vi "GraphWindowGen.vi"() -> (11 "XY Graph":cluster{dbl, dbl}[](graph))   [LabVIEW 2010]
panel:
  out "error out":errorcluster caption="sortie d'erreur"
  in  "error in (no error)":errorcluster
  in  "stop":bool
  in  "ToolsVis":bool=TRUE
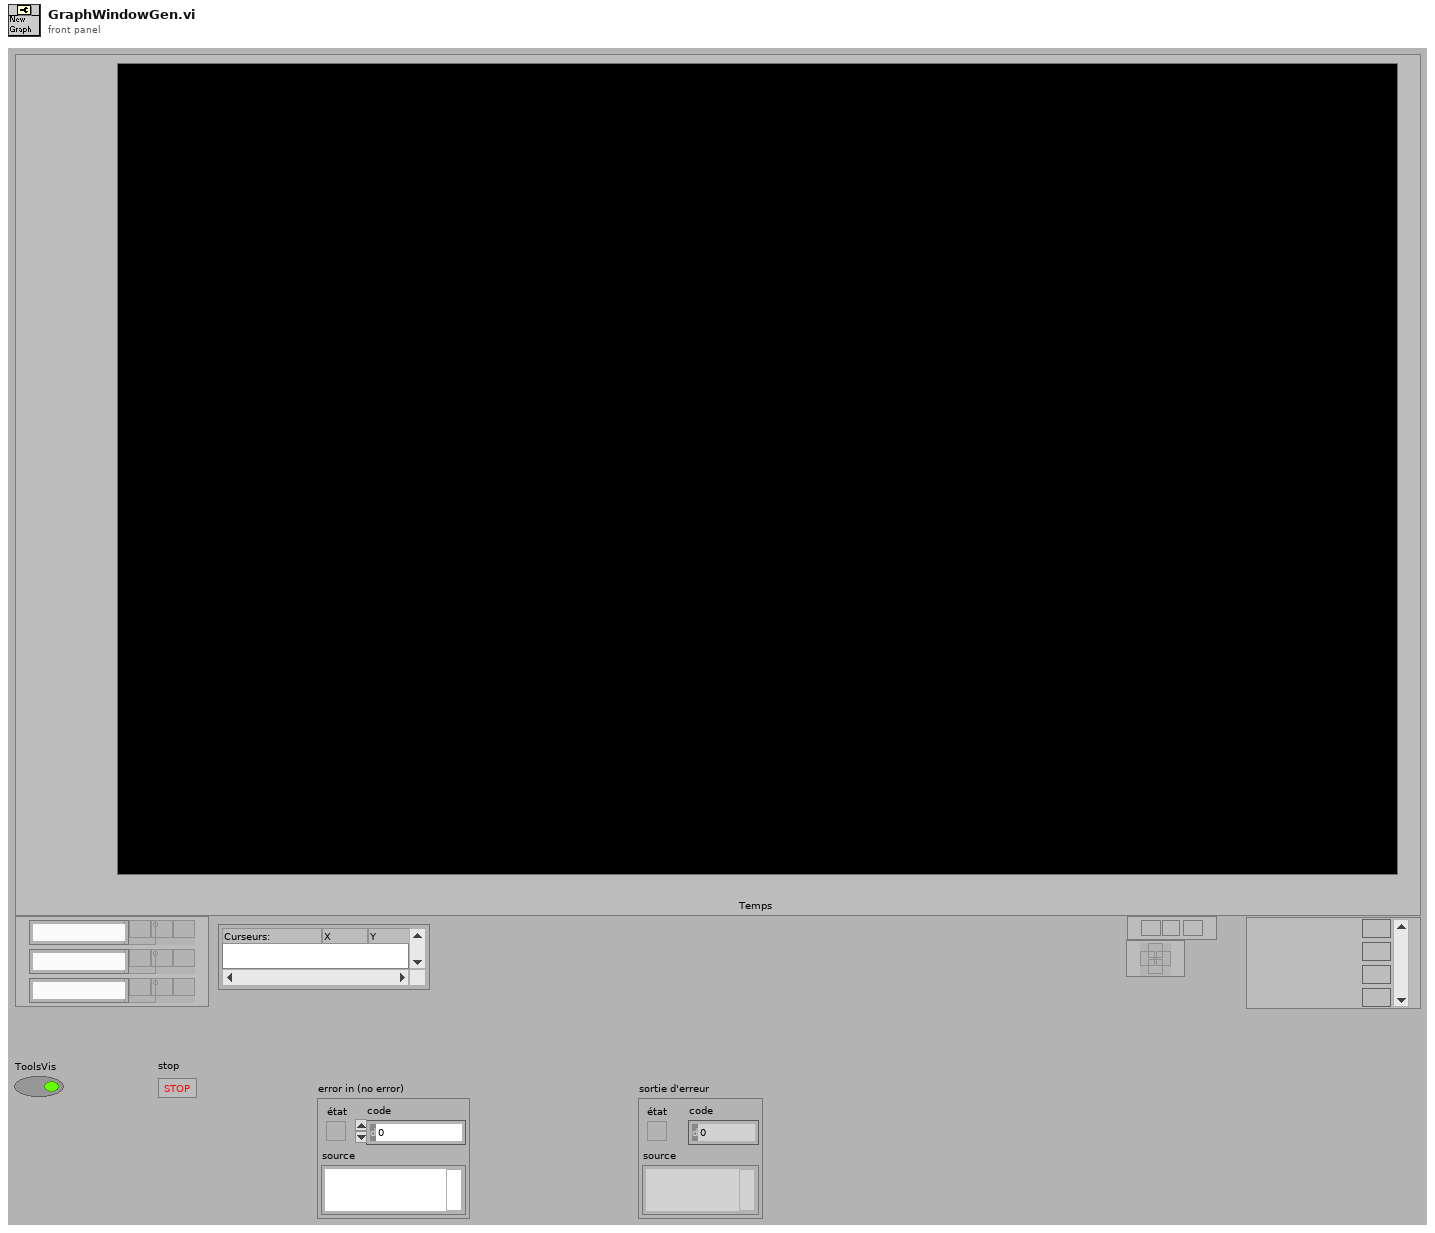
[diagram p1: front panel]
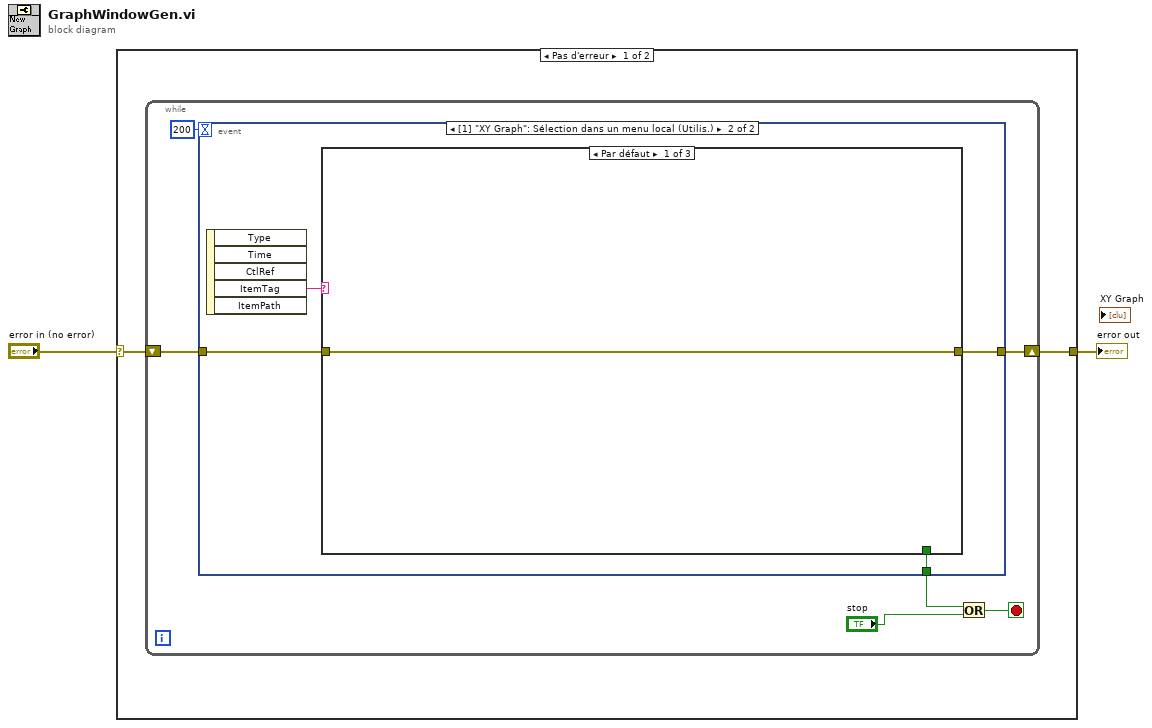
[diagram p0: block diagram]
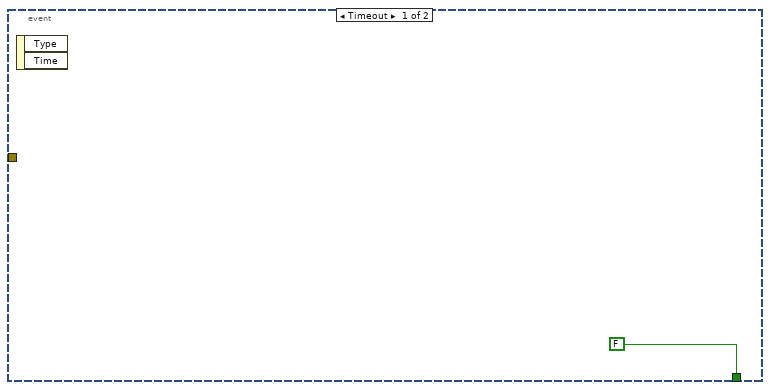
[diagram p2: hidden frame]
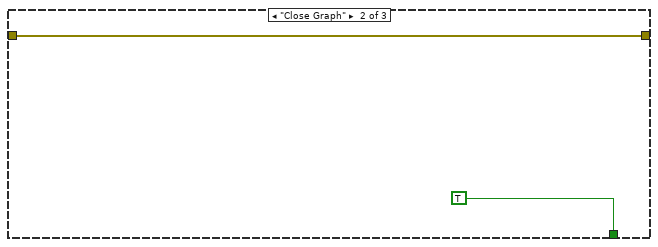
[diagram p3: hidden frame]
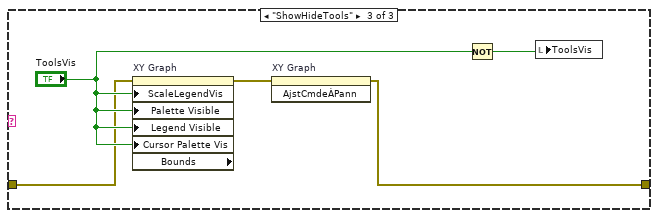
[diagram p4: hidden frame]
diagram:
  n1 = case shown="Pas d'erreur" "error in (no error)" {
    selector: "error in (no error)" -> [w4 w24]
    tunnel: [w3 w24] -> w1
    frame No Error {
      n2 = while {
        shift-right: [w5] -> w3
        shift-left: w4 -> [w6]
        stop <- w8 stop-if-true
        n3 = event shown="[1] \"XY Graph\": Sélection dans un menu local (Utilis.)" {
          selector: _ -> [_ _]
          dyn-events: _ -> [_ _]
          timeout: 200 -> [_ _]
          tunnel: [FALSE w14] -> w9
          tunnel: w6 -> [_ w13]
          tunnel: [_ w12] -> w5
          event Timeout {
            n4 = event-data() -> ()  [unwired: 1 in, 2 out]
          }
          event "XY Graph": Shortcut Menu Selection (User) {
            n5 = event-data() -> ("ItemTag"=w15:string)  [unwired: 1 in, 4 out]
            n6 = case shown="Par défaut" w15 {
              tunnel: [_ TRUE _] -> w14
              tunnel: w13 -> [w16 w17 w20]
              tunnel: [w16 w17 w19] -> w12
              frame Default {
              }
              frame "Close Graph" {
              }
              frame "ShowHideTools" {
                n7 = property on="XY Graph" class="GraphXY (strict)" props=["ScaleLegendVis", "Palette Visible", "Legend Visible", "Cursor Palette Vis", "Bounds"](error in=w20, "ScaleLegendVis"="ToolsVis", "Palette Visible"="ToolsVis", "Legend Visible"="ToolsVis", "Cursor Palette Vis"="ToolsVis") -> (error out=w21:errorcluster)  [unwired: 1 in, 2 out]
                n8 = invoke on="XY Graph" class="GraphXY (strict)" method="AjstCmdeÀPann"(error in=w21) -> (error out=w19:errorcluster)  [unwired: 2 in, 2 out]
                n9 = Not(x="ToolsVis") -> (.not. x?=w23:bool)
                n10 = local write "ToolsVis"(w23) -> ()
              }
            }
          }
        }
        n11 = Or(x=w9, y="stop") -> (x .or. y?=w8:bool)
      }
    }
    frame Error {
    }
  }
  "error out" <- w1
